vi "GlobalPosXbyTime.vi"() -> ()   [LabVIEW 2018]
panel:
  out "Array":dbl[](array[numeric])
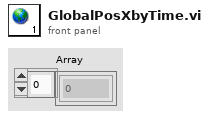
[diagram p1: front panel]
diagram:
